vi "Actor Core.vi"(8 "error in":errorcluster, 11 "Nested in":refnum<class "Servo Motor Emulator.lvclass">) -> (0 "error out":errorcluster, 3 "Actor out":refnum<class "Actor.lvclass">)   [LabVIEW 2020, in "Servo Motor Emulator.lvlib" / "Servo Motor Emulator.lvclass"]
doc: "(<B>Filename</B>: Actor Framework.lvlib:Actor.lvclass:Actor Core.vi)\n\nReceives messages to the actor, reacts to them, and initiates any error handling that may shut the actor down.\n\nDescendant classes may override this VI to append parallel tasks for the actor to complete while it handles messages. Overrides use the Call Parent Method node."
uses:
  Servo Motor Emulator.lvclass
  <vilib>/ActorFramework/Actor/Actor.lvclass
  Servo Motor Emulator.lvclass/Servo Motor Emulator.ctl
  <vilib>/ActorFramework/Stop Msg/Stop Msg.lvclass
  Panel/Panel Messages/Report Temperature and Humidity Msg/Report Temperature and Humidity Msg.lvclass
  C:/Program Files/National Instruments/LabVIEW 2026/vi.lib/ActorFramework/Actor/Actor.lvclass
  C:/Projects/labview_frameworks/actor_framework/Servo Motor Project/Servo Motor Emulator/Servo Motor Emulator.lvclass
  C:/Projects/labview_frameworks/actor_framework/Servo Motor Project/Motor/Motor/Motor.lvclass
  Panel/Panel Messages/Report Humidity Msg/Report Humidity Msg.lvclass
  Panel/Panel Messages/Report Temperature Msg/Report Temperature Msg.lvclass
panel:
  in  "RH":dbl
  in  "Temperature":dbl
  out "Position":dbl(knob) scale=0.0..180.0
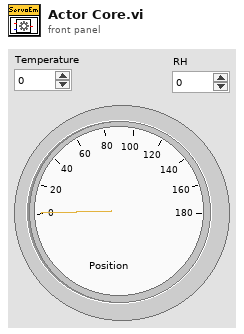
[diagram p1: front panel]
types:
  T1 = cluster{"Stop":refnum<user-event>, "Position":refnum<user-event>}
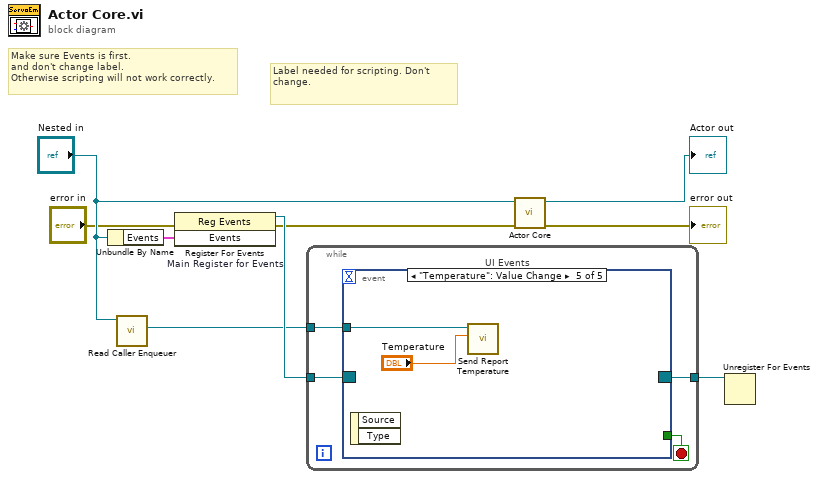
[diagram p0: block diagram]
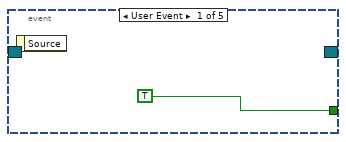
[diagram p2: hidden frame]
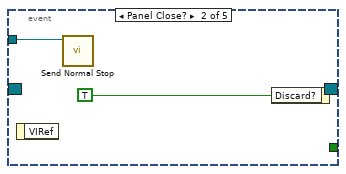
[diagram p3: hidden frame]
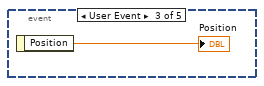
[diagram p4: hidden frame]
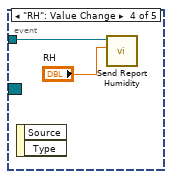
[diagram p5: hidden frame]
diagram:
  # "Label needed for scripting. Don't change."
  # "Make sure Events is first.\nand don't change label.\nOtherwise scripting will not work correctly."
  n1 = Unbundle By Name("Nested in") -> ("Events"=w6:T1)
  n2 = call <vilib>:"Read Caller Enqueuer.vi"("Actor"="Nested in") -> ("Caller Enqueuer"=w3:refnum<class "Message Enqueuer.lvclass">)  [unwired: 10 in]
  n3 = register-events "Main Register for Events"(error in="error in", w6) -> (reference out=w7:refnum<event-registration>, error out=w1:errorcluster)  [unwired: 1 in]
  n4 = while {
    tunnel: w7 -> [w13]
    tunnel: [w11] -> w5
    tunnel: w3 -> [w10]
    stop <- w12 stop-if-true
    n5 = event "UI Events" shown="[4] \"Temperature\": Value Change" {
      selector: w13 -> [_ _ _ _ _]
      dyn-events: [_ _ _ _ _] -> w11
      timeout: _ -> [_ _ _ _ _]
      tunnel: [TRUE _ _ _ _] -> w12
      tunnel: w10 -> [_ w15 _ w19 w21]
      event User Event {
        n6 = event-data() -> ()  [unwired: 1 in, 1 out]
      }
      event Panel Close? {
        n7 = event-data() -> ()  [unwired: 1 in, 1 out]
        n8 = call <vilib>:"Send Normal Stop.vi"("Message Enqueuer"=w15) -> ()  [unwired: 10 in, 1 out]
        n9 = event-data("Discard?"=TRUE) -> ()  [unwired: 1 in, 1 out]
      }
      event User Event {
        n10 = event-data() -> ("Position"=→"Position":dbl)  [unwired: 1 in]
      }
      event "RH": Value Change {
        n11 = event-data() -> ()  [unwired: 1 in, 2 out]
        n12 = call "Send Report Humidity.vi"("Humidity"="RH", "Message Enqueuer"=w19) -> ()  [unwired: 8 in, 2 out]
      }
      event "Temperature": Value Change {
        n13 = event-data() -> ()  [unwired: 1 in, 2 out]
        n14 = call "Send Report Temperature.vi"("Temperature"="Temperature", "Message Enqueuer"=w21) -> ()  [unwired: 8 in, 2 out]
      }
    }
  }
  n15 = call-parent "Actor Core.vi"("error in"=w1, "Actor in"="Nested in") -> ("error out"=→"error out":errorcluster, "Actor out"=→"Actor out":refnum<class "Actor.lvclass">)  [unwired: 8 in]
  n16 = Unregister For Events(event registration refnum=w5) -> ()  [unwired: 1 in, 1 out]
